vi "ResourceVisa_20version.vi"() -> ()   [LabVIEW 2020]
panel:
  out "display file":string
  in  "Path":path
  out "display m3510A":string
  in  "Voltmeter Picotest M3510A":refnum<visa-resource-name>
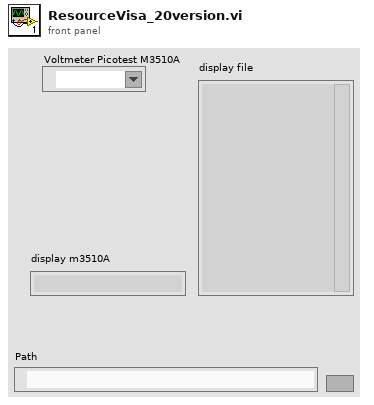
[diagram p1: front panel]
types:
  T1 = enum16{"read/write", "read-only", "write-only", ""}
  T2 = enum16{"open", "replace", "create", "open or create", "replace or create", "replace or create with confirmation", ""}
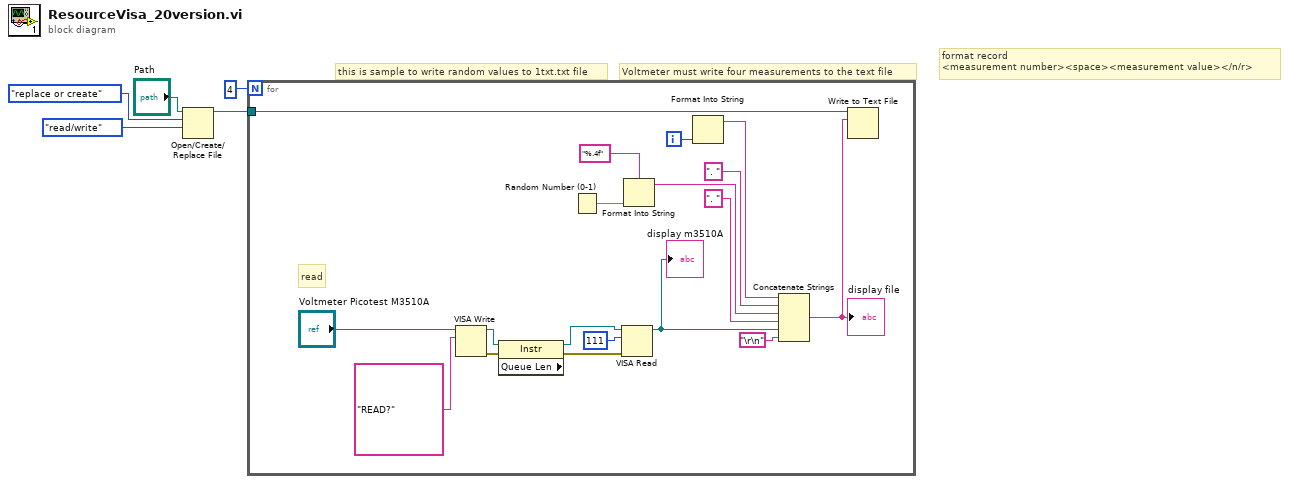
[diagram p0: block diagram]
diagram:
  # "format record \n<measurement number><space><measurement value></n/r>"
  # "Voltmeter must write four measurements to the text file"
  # "this is sample to write random values to 1txt.txt file"
  n1 = Open/Create/Replace File(file path (use dialog)="Path", operation (0:open)=T2."replace or create", access (0:read/write)=T1."read/write") -> (refnum out=w1:refnum<file>)  [unwired: 3 in, 2 out]
  n2 = for {
    N: 4 -> [_]
    tunnel: w1 -> [w15]
    i -> [w14]
    # "read"
    n3 = VISA Write(VISA resource name="Voltmeter Picotest M3510A", write buffer="READ?") -> (VISA resource name out=w20:refnum<visa-resource-name>, error out=w21:errorcluster)  [unwired: 1 in, 1 out]
    n4 = property class="Instr" props=["Queue Len"](reference=w20, error in=w21) -> (reference out=w19:refnum<visa-resource-name>, error out=w18:errorcluster)  [unwired: 1 out]
    n5 = Random Number (0-1)() -> (number: 0 to 1=w16:dbl)
    n6 = VISA Read(VISA resource name=w19, byte count=111, error in (no error)=w18) -> (VISA resource name out=w9:refnum<visa-resource-name>)  [unwired: 3 out]
    "display m3510A" <- w9
    n7 = Format Into String(format string="%.4f", w16) -> (resulting string=w11:string)  [unwired: 2 in, 1 out]
    n8 = Format Into String(w14) -> (resulting string=w13:string)  [unwired: 3 in, 1 out]
    n9 = Concatenate Strings(w13, ". ", w11, ". ", w9, "\r\n") -> (w6:string)
    "display file" <- w6
    n10 = Write to Text File(file (use dialog)=w15, text=w6) -> ()  [unwired: 2 in, 3 out]
  }
